vi "MeaswithZCorr.vi"() -> ()   [LabVIEW 2011]
doc: "This EXAMPLE VI takes a single reading. The data returned includes the reading, timestamp, units, and reading#. Since this is an example, you are free to alter the VI to add addtional elements. Adding or deleting elements will requiore you to modify the VI to separate all of the elements into their individual components."
panel:
  in  "measure time":dbl
  out "Waveform Chart":dbl(graph)
  out "measurement":dbl format="%_8e"
  out "time":string
  out "Read? Output":string
  out "Voltage Output":bool
  in  "Voltage Output\nDisabled/Enable":bool
  in  "Input Voltage":dbl min=0.0 max=100.0 step=0.1
  out "Meter Connect":bool
  in  "Meter Connect\nDisabled/Enable":bool
  out "error out":T1
  in  "GPIB address":string="27"
  in  "error in":T1
  # "Only for current measurements"
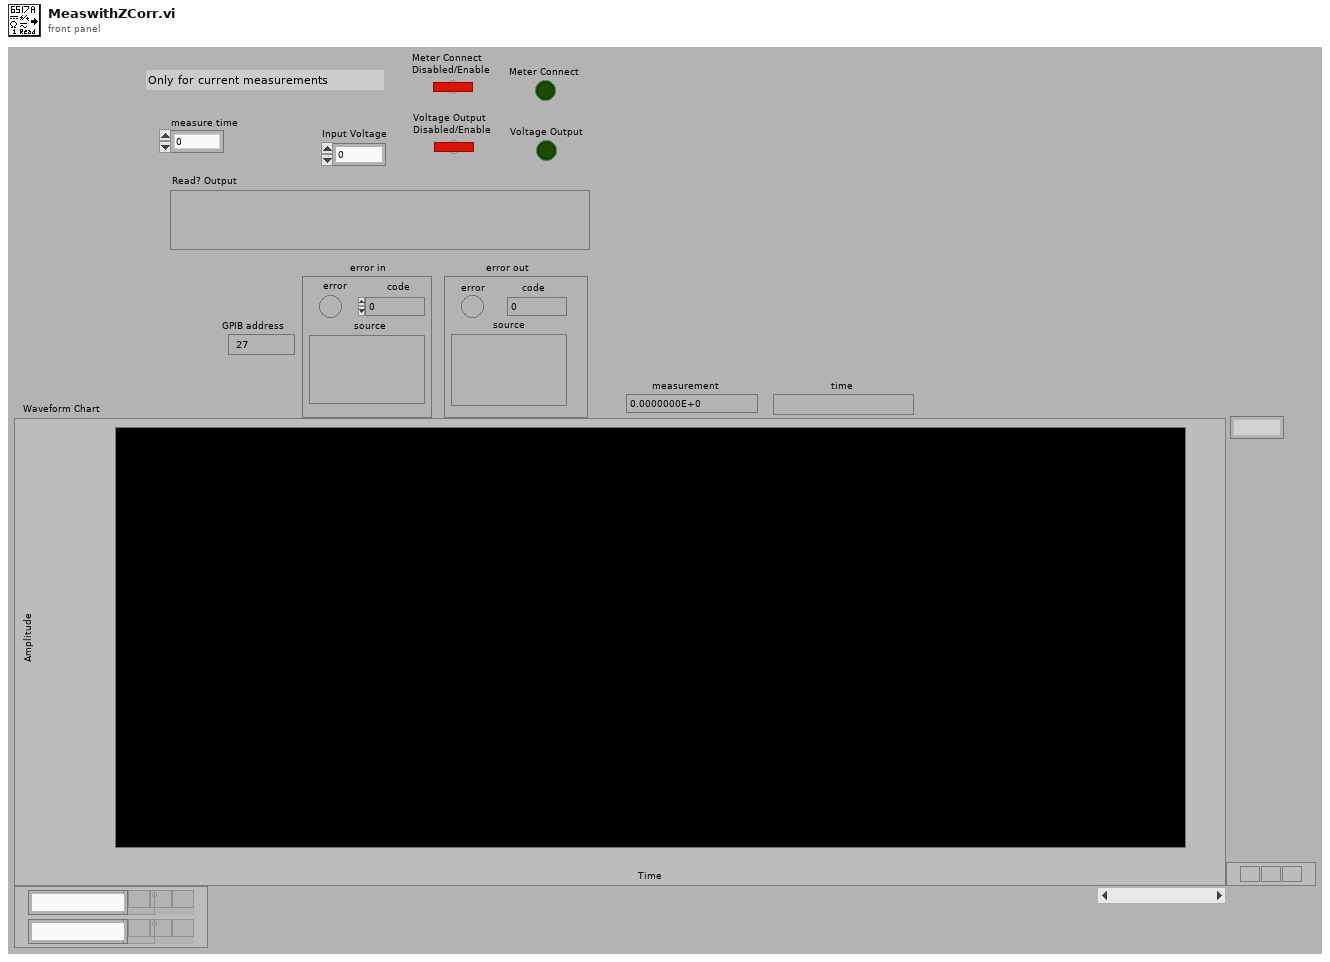
[diagram p1: front panel]
types:
  T1 = cluster{"error":bool, "code":i32, "source":string}
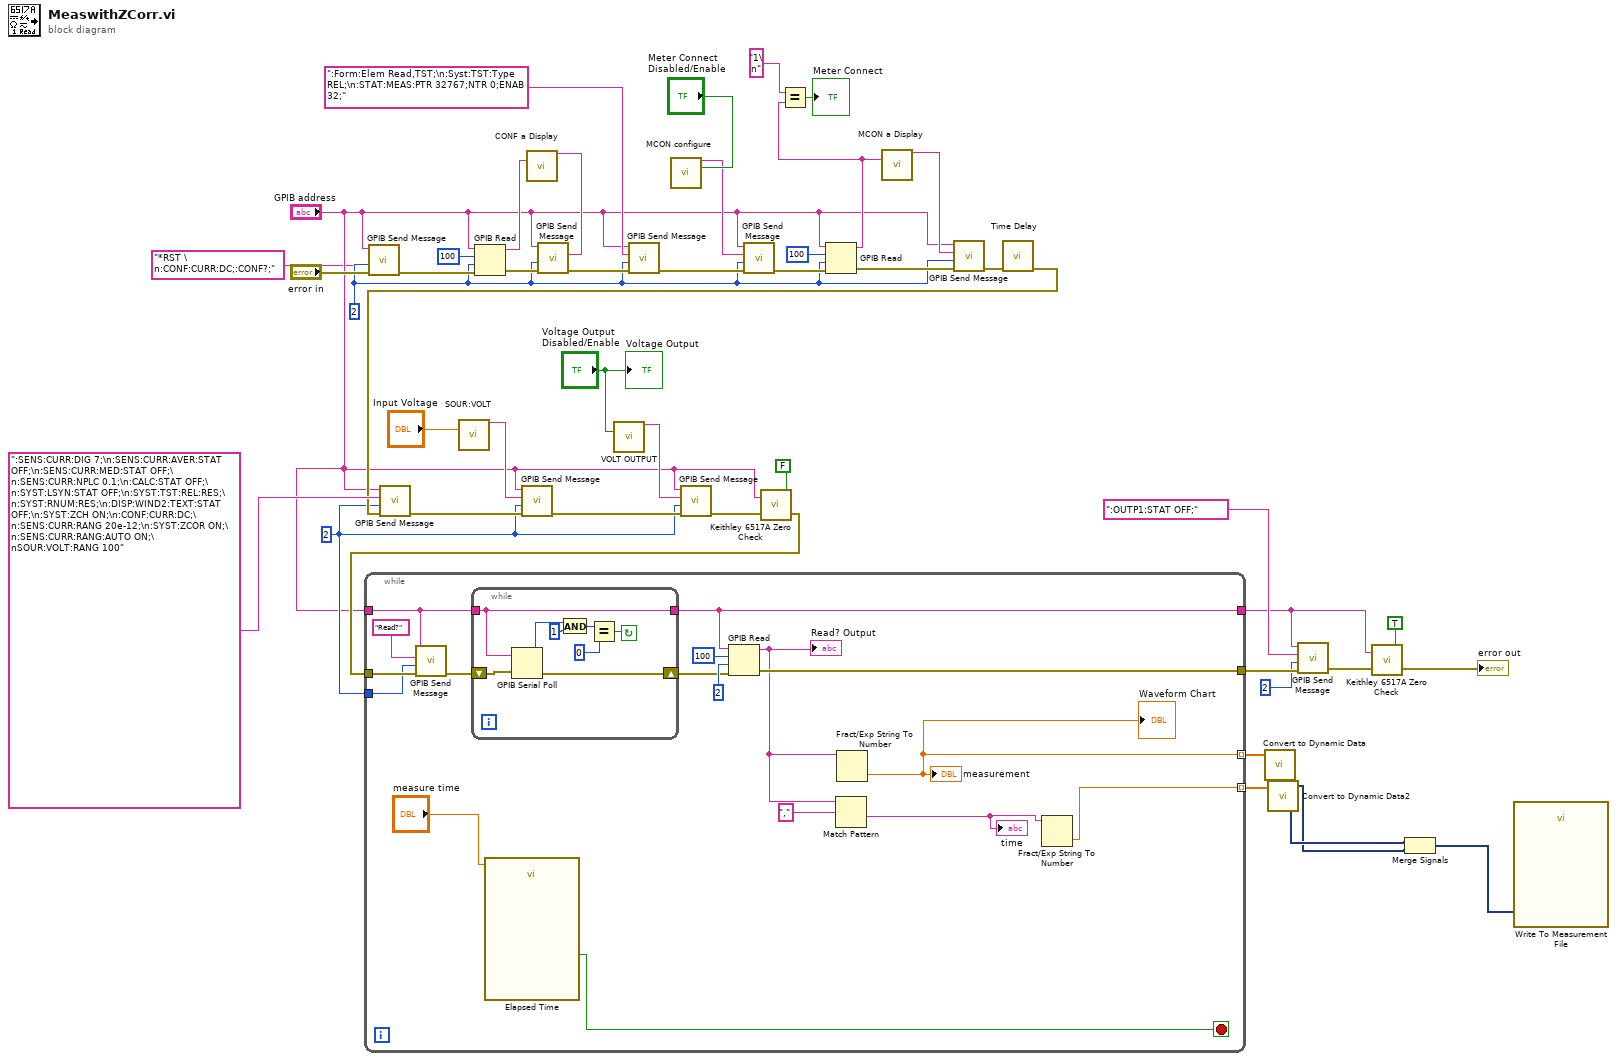
[diagram p0: block diagram]
diagram:
  w15 = 2
  w27 = 2
  n1 = call <instrlib>:"GPIB Send Message.vi"("address string"="GPIB address", "write buffer"="*RST \n:CONF:CURR:DC;:CONF?;", "write mode (set END:0)"=w27, "error in"="error in") -> ("error out"=w41:T1)  [unwired: 3 in, 2 out]
  n2 = call "SOUR:VOLT"("VOLT"="Input Voltage") -> ("Result"=w26:string)  [unwired: 13 in, 1 out]
  n3 = GPIB Read(0:"GPIB address", 1:100, 2:w27, 3:w41) -> (5:w42:string, 7:w44:errorcluster)  [unwired: 1 in, 1 out]
  n4 = call "CONF a Display"("VAR"=w42) -> ("Result"=w43:string)  [unwired: 13 in, 1 out]
  n5 = call <instrlib>:"GPIB Send Message.vi"("address string"="GPIB address", "write buffer"=w43, "write mode (set END:0)"=w27, "error in"=w44) -> ("error out"=w39:T1)  [unwired: 3 in, 2 out]
  n6 = call "VOLT OUTPUT"("VOLTOUTPUT"="Voltage Output\nDisabled/Enable") -> ("Result"=w23:string)  [unwired: 13 in, 1 out]
  n7 = call <instrlib>:"GPIB Send Message.vi"("address string"="GPIB address", "write buffer"=":Form:Elem Read,TST;\n:Syst:TST:Type REL;\n:STAT:MEAS:PTR 32767;NTR 0;ENAB 32;", "write mode (set END:0)"=w27, "error in"=w39) -> ("error out"=w35:T1)  [unwired: 3 in, 2 out]
  n8 = call "MCON configure"("MCON"="Meter Connect\nDisabled/Enable") -> ("Result"=w36:string)  [unwired: 13 in, 1 out]
  n9 = call <instrlib>:"GPIB Send Message.vi"("address string"="GPIB address", "write buffer"=w36, "write mode (set END:0)"=w27, "error in"=w35) -> ("error out"=w34:T1)  [unwired: 3 in, 2 out]
  n10 = GPIB Read(0:"GPIB address", 1:100, 2:w27, 3:w34) -> (5:w31:string, 7:w30:errorcluster)  [unwired: 1 in, 1 out]
  n11 = Equal?(x="1\n", y=w31) -> (x = y?=→"Meter Connect":bool)
  n12 = call "MCON a Display"("VAR2"=w31) -> ("Result"=w29:string)  [unwired: 13 in, 1 out]
  n13 = call <instrlib>:"GPIB Send Message.vi"("address string"="GPIB address", "write buffer"=w29, "write mode (set END:0)"=w27, "error in"=w30) -> ("error out"=w28:T1)  [unwired: 3 in, 2 out]
  n14 = call "Time Delay"("error in (no error)"=w28) -> ("error out"=w19:errorcluster)  [unwired: 10 in]
  n15 = call <instrlib>:"GPIB Send Message.vi"("address string"="GPIB address", "write buffer"=":SENS:CURR:DIG 7;\n:SENS:CURR:AVER:STAT OFF;\n:SENS:CURR:MED:STAT OFF;\n:SENS:CURR:NPLC 0.1;\n:CALC:STAT OFF;\n:SYST:LSYN:STAT OFF;\n:SYST:TST:REL:RES;\n:SYST:RNUM:RES;\n:DISP:WIND2:TEXT:STAT OFF;\n:SYST:ZCH ON;\n:CONF:CURR:DC;\n:SENS:CURR:RANG 20e-12;\n:SYST:ZCOR ON;\n:SENS:CURR:RANG:AUTO ON;\nSOUR:VOLT:RANG 100", "write mode (set END:0)"=w15, "error in"=w19) -> ("error out"=w21:T1)  [unwired: 3 in, 2 out]
  n16 = call <instrlib>:"GPIB Send Message.vi"("address string"="GPIB address", "write buffer"=w26, "write mode (set END:0)"=w15, "error in"=w21) -> ("error out"=w20:T1)  [unwired: 3 in, 2 out]
  n17 = call <instrlib>:"GPIB Send Message.vi"("address string"="GPIB address", "write buffer"=w23, "write mode (set END:0)"=w15, "error in"=w20) -> ("error out"=w17:T1)  [unwired: 3 in, 2 out]
  n18 = call <instrlib>:"Keithley 6517A Zero Check.vi"("Zero Check"=FALSE, "error in"=w17, "GPIB address"="GPIB address") -> ("error out"=w16:T1)
  n19 = while {
    tunnel: w16 -> [w63]
    tunnel: w15 -> [w61]
    tunnel: "GPIB address" -> [w58]
    tunnel: [w55] -> w12
    tunnel: [w54] -> w1
    tunnel: [w49] -> w7 mode=indexing
    tunnel: [w50] -> w6 mode=indexing
    stop <- w53 stop-if-true
    n20 = call <instrlib>:"GPIB Send Message.vi"("address string"=w58, "write buffer"="Read?", "write mode (set END:0)"=w61, "error in"=w63) -> ("error out"=w57:T1)  [unwired: 3 in, 2 out]
    n21 = while {
      tunnel: w58 -> [w64]
      shift-right: [w65] -> w56
      shift-left: w57 -> [w66]
      tunnel: [w64] -> w54
      stop <- w70 continue-if-true
      n22 = GPIB Serial Poll(0:w64, 1:w66) -> (2:w69:i16, 4:w65:errorcluster)  [unwired: 1 out]
      n23 = And(x=w69, y=1) -> (x .and. y?=w67:i32)
      n24 = Equal?(x=w67, y=0) -> (x = y?=w70:bool)
    }
    n25 = call "Elapsed Time"("Time Target (s)"="measure time") -> ("Time has Elapsed"=w53:bool)  [unwired: 11 in, 7 out]
    n26 = GPIB Read(0:w54, 1:100, 2:2, 3:w56) -> (5:w52:string, 7:w55:errorcluster)  [unwired: 1 in, 1 out]
    "Read? Output" <- w52
    n27 = Match Pattern(string=w52, regular expression=",") -> (after substring=w48:string)  [unwired: 1 in, 3 out]
    "time" <- w48
    n28 = Fract/Exp String To Number(string=w52) -> (number=w49:dbl)  [unwired: 3 in, 1 out]
    "measurement" <- w49
    "Waveform Chart" <- w49
    n29 = Fract/Exp String To Number(string=w48) -> (number=w50:dbl)  [unwired: 3 in, 1 out]
  }
  n30 = call "Convert to Dynamic Data"("Array"=w7) -> ("Dynamic Data Type"=w4:dynamicdata)  [unwired: 3 in]
  n31 = call "Convert to Dynamic Data2"("Array"=w6) -> ("Dynamic Data Type"=w3:dynamicdata)  [unwired: 3 in]
  n32 = call <instrlib>:"GPIB Send Message.vi"("address string"=w1, "write buffer"=":OUTP1:STAT OFF;", "write mode (set END:0)"=2, "error in"=w12) -> ("error out"=w10:T1)  [unwired: 3 in, 2 out]
  n33 = call <instrlib>:"Keithley 6517A Zero Check.vi"("Zero Check"=TRUE, "error in"=w10, "GPIB address"=w1) -> ("error out"=→"error out":T1)
  n34 = Merge Signals(w4, w3) -> (w2:dynamicdata)
  n35 = call "Write To Measurement File"("Signals"=w2) -> ()  [unwired: 16 in, 3 out]
  "Voltage Output" <- "Voltage Output\nDisabled/Enable"
